vi "ExSubSaveMultiFrame.vi"(0 "Number of Images":u32, 1 "Display Handle":u32, 2 "file handle":u32, 3 "error in (no error)":errorcluster, 4 "Data handles":u32[](array[numeric])) -> (5 "Display Handle":u32, 6 "file Handle":u32, 7 "error out":errorcluster)   [LabVIEW 2010]
panel:
  # "ExSubSaveMultiFrame.vi :this sub vi takes an array of image handles\nand displays and saves them. user may want to put a delay in loop so that \nall images are seen."
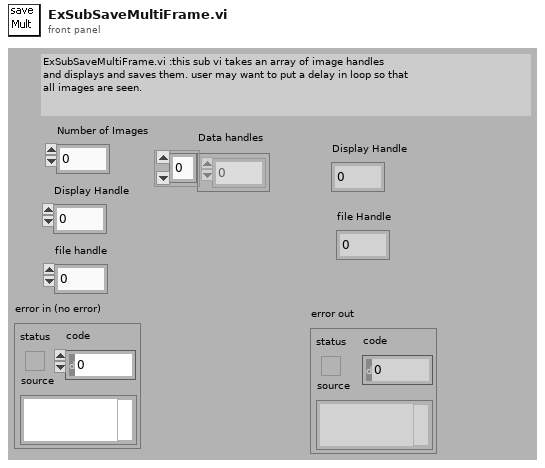
[diagram p1: front panel]
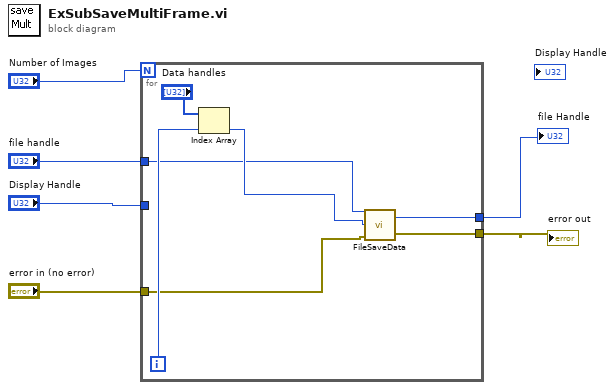
[diagram p0: block diagram]
diagram:
  n1 = for {
    N: "Number of Images" -> [_]
    tunnel: "Display Handle" -> [_]
    tunnel: "file handle" -> [w10]
    tunnel: "error in (no error)" -> [w7]
    tunnel: [w9] -> w2
    tunnel: [w8] -> w1
    i -> [w13]
    n2 = Index Array(array="Data handles", index=w13) -> (element=w11:u32)
    n3 = call <userlib>:"FileSaveData.vi"("error in"=w7, "Image Handle"=w11, "File Handle"=w10) -> ("error out"=w9:errorcluster, "File Handle"=w8:u32)
  }
  "error out" <- w2
  "file Handle" <- w1
